vi "Read.vi"(4 "Com Port":refnum<visa-resource-name>) -> (0 "Ch 2 out":dbl format="%.6f", 1 "Com out":refnum<visa-resource-name>, 2 "Ch 1 out":dbl format="%.6f", 6 "String":string)   [LabVIEW 2020]
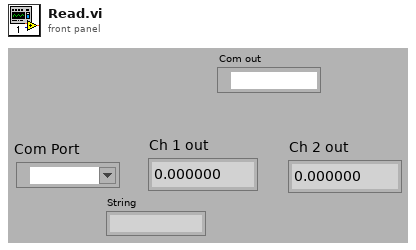
[diagram p1: front panel]
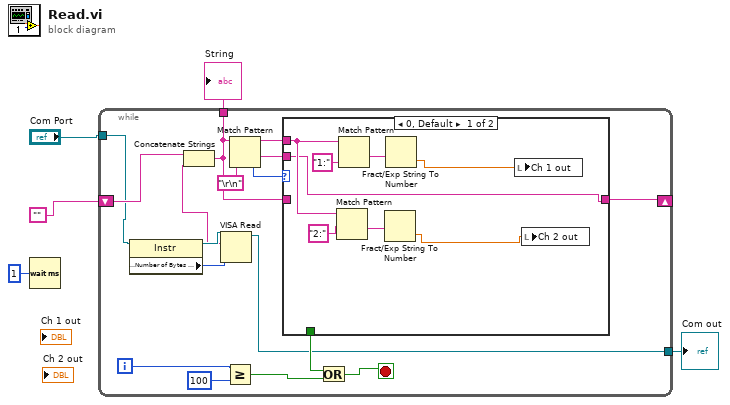
[diagram p0: block diagram]
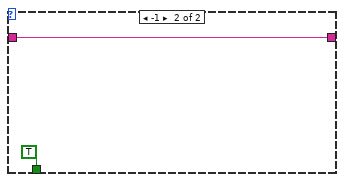
[diagram p2: hidden frame]
diagram:
  n1 = Wait (ms)(milliseconds to wait=u32 1) -> ()  [unwired: 1 out]
  n2 = while {
    shift-right: [w21] -> _
    shift-left: "" -> [w18]
    tunnel: "Com Port" -> [w16]
    tunnel: [w7] -> w2
    tunnel: [w6] -> w1
    i -> [w9]
    stop <- w10 stop-if-true
    n3 = property class="Instr"(reference=w16) -> (reference out=w15:refnum<visa-resource-name>, "Serial Settings:Number of Bytes at Serial Port"=w14:u32)  [unwired: 1 in, 1 out]
    n4 = VISA Read(VISA resource name=w15, byte count=w14) -> (VISA resource name out=w7:refnum<visa-resource-name>, read buffer=w13:string)  [unwired: 1 in, 2 out]
    n5 = Concatenate Strings(w18, w13) -> (w6:string)
    n6 = Greater Or Equal?(x=w9, y=i16 100 ("x")) -> (x >= y?=w12:bool)
    n7 = Match Pattern(string=w6, regular expression="\r\n") -> (before substring=w19:string, after substring=w20:string, offset past match=w22:i32)  [unwired: 1 in, 1 out]
    n8 = case shown="0, Default" w22 {
      tunnel: [w23 w33] -> w21
      tunnel: w6 -> [_ w33]
      tunnel: w20 -> [w23 _]
      tunnel: w19 -> [w28 _]
      tunnel: [TRUE ("x") TRUE ("x")] -> w11
      frame 0, Default {
        n9 = Match Pattern(string=w28, regular expression="2:") -> (after substring=w27:string)  [unwired: 1 in, 3 out]
        n10 = Match Pattern(string=w28, regular expression="1:") -> (after substring=w26:string)  [unwired: 1 in, 3 out]
        n11 = Fract/Exp String To Number(string=w27) -> (number=w24:dbl)  [unwired: 3 in, 1 out]
        n12 = Fract/Exp String To Number(string=w26) -> (number=w25:dbl)  [unwired: 3 in, 1 out]
        n13 = local write "Ch 1 out"(w25) -> ()
        n14 = local write "Ch 2 out"(w24) -> ()
      }
      frame -1 {
      }
    }
    n15 = Or(x=w11, y=w12) -> (x .or. y?=w10:bool)
  }
  "Com out" <- w2
  "String" <- w1
